vi "test_CalculateSpecificationBuildOrder_TargetsDifferentCompilersAdvancedPPLSolution.vi"() -> (3 "Pass?":bool)   [LabVIEW 2019, in "Tests.SolutionBuilder.lvlib"]
uses:
  Tests.SolutionBuilder.lvlib
  SolutionBuilder/SolutionBuilder.lvclass
  SolutionBuilder/ProjectItem/ProjectItem.lvclass
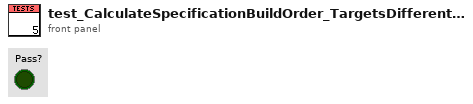
[diagram p1: front panel]
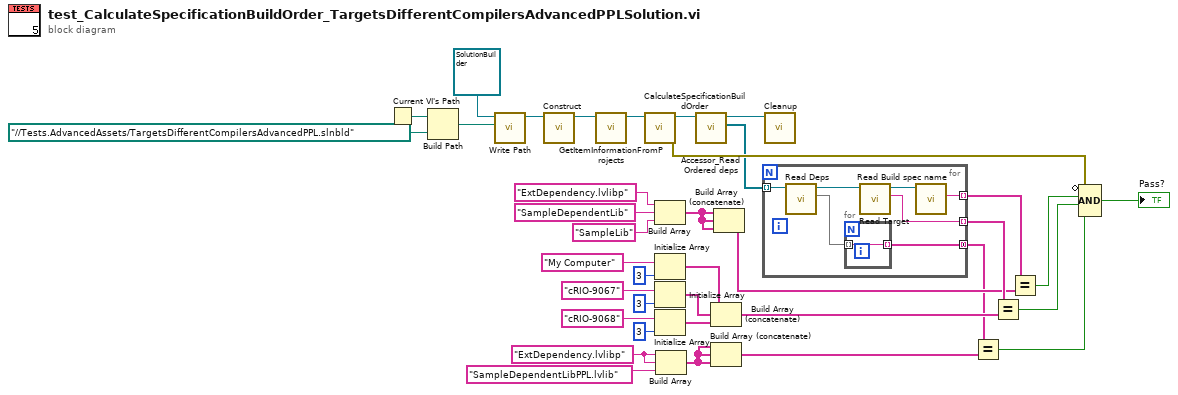
[diagram p0: block diagram]
diagram:
  w7 = "ExtDependency.lvlibp" ("Build spec name")
  n1 = Current VI's Path() -> (path=w36:path)
  n2 = Build Path(base path=w36, name or relative path=path "../../Tests.AdvancedAssets/TargetsDifferentCompilersAdvancedPPL.slnbld" ("Path")) -> (appended path=w34:path)
  n3 = call "Write Path.vi"("Path"=w34, "SolutionBuilder in"=refnum<class "SolutionBuilder.lvclass"> refnum) -> ("SolutionBuilder out"=w33:refnum<class "SolutionBuilder.lvclass">)  [unwired: 9 in]
  n4 = call "Construct.vi"("SolutionBuilder in"=w33) -> ("SolutionBuilder out"=w31:refnum<class "SolutionBuilder.lvclass">)  [unwired: 9 in, 1 out]
  n5 = call "GetItemInformationFromProjects.vi"("SolutionBuilder in"=w31) -> ("SolutionBuilder out"=w30:refnum<class "SolutionBuilder.lvclass">)  [unwired: 9 in, 1 out]
  n6 = call "CalculateSpecificationBuildOrder.vi"("SolutionBuilder in"=w30) -> ("error out"=w27:errorcluster, "SolutionBuilder out"=w29:refnum<class "SolutionBuilder.lvclass">)  [unwired: 9 in]
  n7 = Build Array("ExtDependency.lvlibp" ("Build spec name"), "SampleDependentLib" ("Build spec name"), "SampleLib" ("Build spec name")) -> (w9:string[])
  n8 = Initialize Array("My Computer" ("Build spec name"), 3 ("dimension size")) -> (w18:string[])
  n9 = Initialize Array("cRIO-9067" ("Build spec name"), 3 ("dimension size")) -> (w17:string[])
  n10 = Initialize Array("cRIO-9068" ("Build spec name"), 3 ("dimension size")) -> (w16:string[])
  n11 = Build Array(w7, w7, "SampleDependentLibPPL.lvlib" ("Build spec name")) -> (w5:string[])
  n12 = call "Accessor_Read Ordered deps.vi"("SolutionBuilder in"=w29) -> ("Ordered deps"=w26:refnum<class "ProjectItem.lvclass">[], "SolutionBuilder out"=w28:refnum<class "SolutionBuilder.lvclass">)  [unwired: 8 in, 1 out]
  n13 = Build Array (concatenate)(w18, w17, w16) -> (w13:string[])
  n14 = Build Array (concatenate)(w5, w5, w5) -> (w3:string[])
  n15 = Build Array (concatenate)(w9, w9, w9) -> (w8:string[])
  n16 = for {
    tunnel: w26 -> [w40] mode=indexing
    tunnel: [w44] -> w25 mode=indexing
    tunnel: [w42] -> w15 mode=indexing
    tunnel: [w38] -> w4 mode=concatenating
    n17 = call "Read Deps.vi"("ProjectItem in"=w40) -> ("Deps"=w41:set{string}, "ProjectItem out"=w39:refnum<class "ProjectItem.lvclass">)  [unwired: 9 in]
    n18 = for {
      tunnel: w41 -> [w45] mode=indexing
      tunnel: [w45] -> w38 mode=indexing
    }
    n19 = call "Read Target.vi"("ProjectItem in"=w39) -> ("Target"=w42:string, "ProjectItem out"=w43:refnum<class "ProjectItem.lvclass">)  [unwired: 9 in]
    n20 = call "Read Build spec name.vi"("ProjectItem in"=w43) -> ("Build spec name"=w44:string)  [unwired: 9 in, 1 out]
  }
  n21 = call "Cleanup.vi"("SolutionBuilder in"=w28) -> ()  [unwired: 9 in, 2 out]
  n22 = Equal?(x=w4, y=w3) -> (x = y?=w2:bool)
  n23 = Equal?(x=w15, y=w13) -> (x = y?=w14:bool)
  n24 = Equal?(x=w25, y=w8) -> (x = y?=w32:bool)
  n25 = Compound Arithmetic op=AND(invert w27, w32, w14, w2) -> (→"Pass?":bool)
